vi "GUI Recalculate.vi"(11 "FFmeter settings":T1={"AC Source"={"AC Source type"=enum."Fluke 5XXX calibrator", "VISA"="", "Ref. clock (Hz)"=0.0, "status ref"=refnum}, "TWM pipe"="\\\\.\\pipe\\TWM:server", "Measurement status ref"=refnum, "TWM Status ref"=refnum, "Abort ref"=refnum, "DC meter"={"DC meter type"=enum."H/A/K 3458", "DC meter VISA"="", "NPLC"=10, "No of readings"=3, "status ref"=refnum}, "Measurement properties"={"Measurement frequencies (Hz)"=[1000.0], "Sampling frequency (Hz)"=500000.0, "Signal amplitude (V)"=4.5, "AC-DC settle time (s)"=20.0, "Record length (multiples of period)"=[1000.0, 10000.0, 1000.0], "Measurement template file"=path "", "Row of START keyword"=0, "Row of STOP keyword"=0, "Calculate RMS from samples"=FALSE, "AC-DC warm up time (s)"=300.0, "Measurement template line"=[]}, "Skip waiting ref"=refnum, "Octave paths"={"GNU Octave path"=path "C:/Program Files/GNU Octave/Octave-6.2.0/mingw64/bin", "TWM+QWTB path"=path "C:/Users/labina/Desktop/TWM-1.8.7.0-full/octprog", "lvlib path"=path "D:/martin/WAC/WACsw - github/control_software/Filter function meter/external libraries/GOLPI 0.7.3.1 source distribution LV 20.0 32 bit/lv_proc.dll"}} {"Measurement properties"."Record length (multiples of period)" format="%#_3p"; "Measurement properties"."Sampling frequency (Hz)" format="%#_3p"; "Measurement properties"."Measurement frequencies (Hz)" format="%#_3p"}) -> (3 "FFmeter settings out":T1={"AC Source"={"AC Source type"=enum."Fluke 5XXX calibrator", "VISA"="", "Ref. clock (Hz)"=0.0, "status ref"=refnum}, "TWM pipe"="\\\\.\\pipe\\TWM:server", "Measurement status ref"=refnum, "TWM Status ref"=refnum, "Abort ref"=refnum, "DC meter"={"DC meter type"=enum."H/A/K 3458", "DC meter VISA"="", "NPLC"=10, "No of readings"=3, "status ref"=refnum}, "Measurement properties"={"Measurement frequencies (Hz)"=[1000.0], "Sampling frequency (Hz)"=500000.0, "Signal amplitude (V)"=4.5, "AC-DC settle time (s)"=20.0, "Record length (multiples of period)"=[1000.0, 10000.0, 1000.0], "Measurement template file"=path "", "Row of START keyword"=0, "Row of STOP keyword"=0, "Calculate RMS from samples"=FALSE, "AC-DC warm up time (s)"=300.0, "Measurement template line"=[]}, "Skip waiting ref"=refnum, "Octave paths"={"GNU Octave path"=path "C:/Program Files/GNU Octave/Octave-6.2.0/mingw64/bin", "TWM+QWTB path"=path "C:/Users/labina/Desktop/TWM-1.8.7.0-full/octprog", "lvlib path"=path "D:/martin/WAC/WACsw - github/control_software/Filter function meter/external libraries/GOLPI 0.7.3.1 source distribution LV 20.0 32 bit/lv_proc.dll"}} {"Measurement properties"."Record length (multiples of period)" format="%#_3p"; "Measurement properties"."Sampling frequency (Hz)" format="%#_3p"; "Measurement properties"."Measurement frequencies (Hz)" format="%#_3p"})   [LabVIEW 2020]
doc: "Use this template to build a producer/consumer design pattern with events to produce queue items. Use this design pattern instead of the User Interface Event Handler pattern for user interfaces when you want to execute code asynchronously in response to an event without slowing the user interface responsiveness."
uses:
  GUI/Type definitions/FFmeter settings.ctl
  General AC source/Type definitions/AC Source.ctl
  General AC source/Type definitions/AC Source type.ctl
  General DC meter/Type definitions/DC meter.ctl
  General DC meter/Type definitions/DC meter type.ctl
  Measurement/Type definitions/Measuement properties.ctl
  <vilib>/Utility/NIReport.llb/Report Type.ctl
  external libraries/GOLPI 0.7.3.1 source distribution LV 20.0 32 bit/GOLPI reference Type Def.ctl
  external libraries/GOLPI 0.7.3.1 source distribution LV 20.0 32 bit/Pipe Handle.ctl
  <vilib>/Utility/error.llb/Error Cluster From Error Code.vi
  <vilib>/ErrorRing/Error Ring.xnode
  <vilib>/addons/_office/excel.llb/Excel Get Data ([str]).vi
  external libraries/varilib/varilib.lvlib
  <vilib>/addons/_office/NI_ReportGenerationToolkit.lvlib
  <vilib>/Utility/NIReport.llb/NI_report.lvclass
  <vilib>/Utility/NIReport.llb/NI_ReportGenerationCore.lvlib
  external libraries/GOLPI 0.7.3.1 source distribution LV 20.0 32 bit/LV Process library.lvlib
  external libraries/GOLPI 0.7.3.1 source distribution LV 20.0 32 bit/GOLPI library.lvlib
  <vilib>/Utility/NIReport.llb/Excel/NI_Excel.lvclass
panel:
  out "Progress":i32(slide) min=0 max=3 scale=0.0..10.0
  in  "TWM+QWTB path":path=path "C:/Users/labina/Desktop/TWM-1.8.7.0-full/octprog"
  in  "GNU Octave path":path=path "C:/Program Files/GNU Octave/Octave-6.2.0/mingw64/bin"
  out "gui_elements":refnum<vi>[](array[refnum])
  in  "OK":bool
  in  "cancel":bool
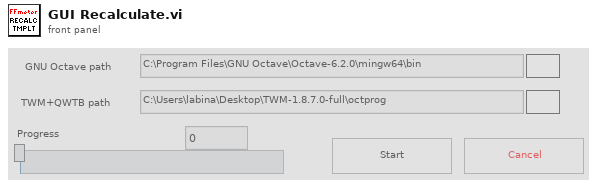
[diagram p1: front panel]
types:
  T1 = typedef "FFmeter settings.ctl" = cluster{"AC Source":T2, "TWM pipe":string, "Measurement status ref":refnum<vi>, "TWM Status ref":refnum<vi>, "Abort ref":refnum<vi>, "DC meter":T4, "Measurement properties":T6, "Skip waiting ref":refnum<vi>, "Octave paths":cluster{"GNU Octave path":path, "TWM+QWTB path":path, "lvlib path":path}}
  T2 = typedef "AC Source.ctl" = cluster{"AC Source type":T3, "VISA":refnum<visa-resource-name>, "Ref. clock (Hz)":dbl, "status ref":refnum<vi>}
  T3 = typedef "AC Source type.ctl" = enum16{"Fluke 5XXX calibrator", "Tektronix AFG3101C", "dummy"}
  T4 = typedef "DC meter.ctl" = cluster{"DC meter type":T5, "DC meter VISA":refnum<visa-resource-name>, "NPLC":i32, "No of readings":i32, "status ref":refnum<vi>}
  T5 = typedef "DC meter type.ctl" = enum16{"H/A/K 3458", "FLuke 8508A", "dummy"}
  T6 = typedef "Measuement properties.ctl" = cluster{"Measurement frequencies (Hz)":dbl[], "Sampling frequency (Hz)":dbl, "Signal amplitude (V)":dbl, "AC-DC settle time (s)":dbl, "Record length (multiples of period)":dbl[], "Measurement template file":path, "Row of START keyword":i32, "Row of STOP keyword":i32, "Calculate RMS from samples":bool, "AC-DC warm up time (s)":dbl, "Measurement template line":i32[]}
  T7 = typedef "GOLPI library.lvlib/GOLPI reference Type Def.ctl" = cluster{"pipe handle":T8, "fast read timeout [ms]":u32, "fast read settle time [ms]":u32, "fast read to multiple [ms]":u32, "max elements per input line":u32, "slow read timeout [ms]":u32, "stdin double format specifier":string, "max elements per stdout output column":u32, "console mode bitstream":bool, "bitstream first read timeout [ms]":u32, "bitstream read timeout [ms]":u32, "struct transfer possible":bool, "matlab mode":bool}
  T8 = typedef "LV Process library.lvlib/Pipe Handle.ctl" = cluster{"lv_proc.dll file path":path, "process instance handle":u32[], "debug mode":bool, "debug data":cluster{"time":timestamp, "stdin":bool, "data":string}[]}
  T9 = enum16{"maximized", "minimized", "normal", "no change"}
  T10 = typedef "NI_ReportGenerationCore.lvlib/Report Type.ctl" = enum16{"HTML", "Word", "Excel"}
  T11 = cluster{"GNU Octave path":path, "TWM+QWTB path":path, "lvlib path":path}
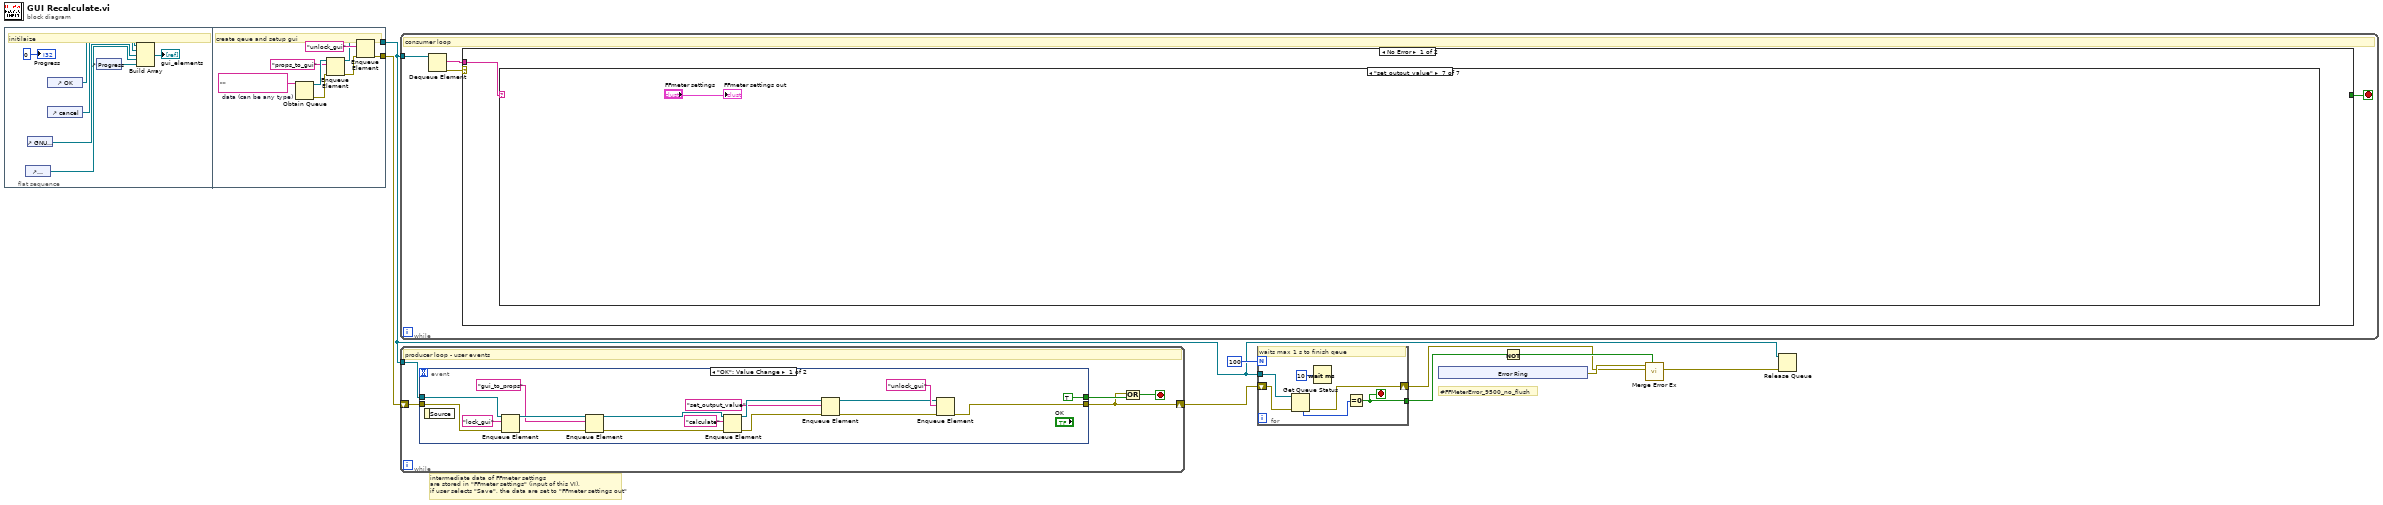
[diagram p0: block diagram]
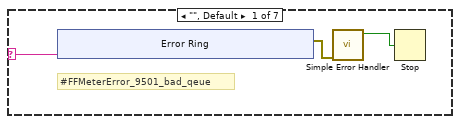
[diagram p2: hidden frame]
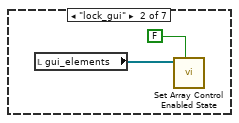
[diagram p3: hidden frame]
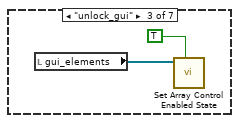
[diagram p4: hidden frame]
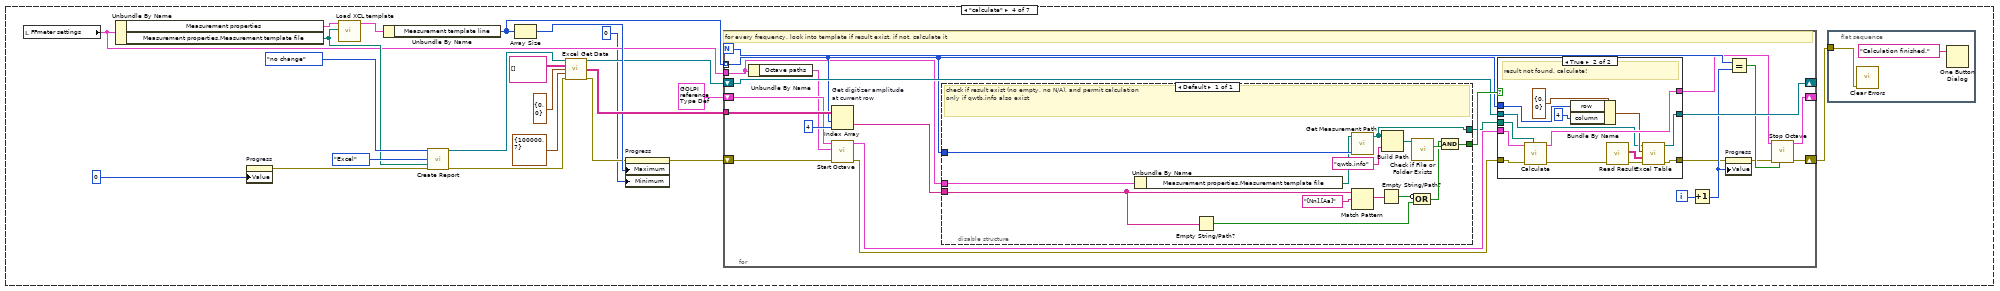
[diagram p5: hidden frame]
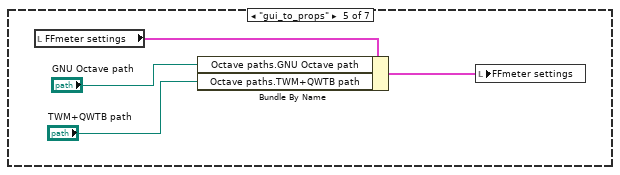
[diagram p7: hidden frame]
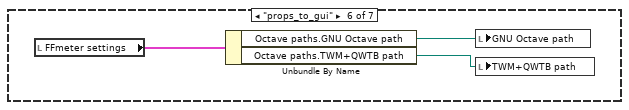
[diagram p8: hidden frame]
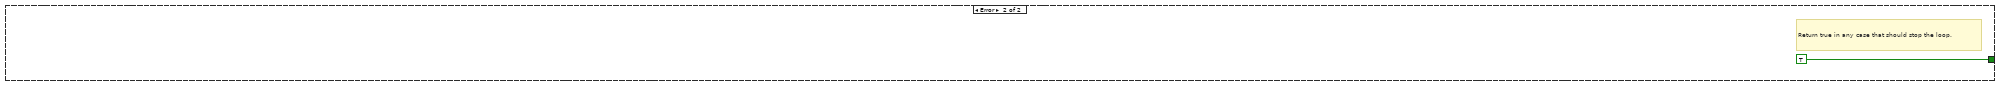
[diagram p9: hidden frame]
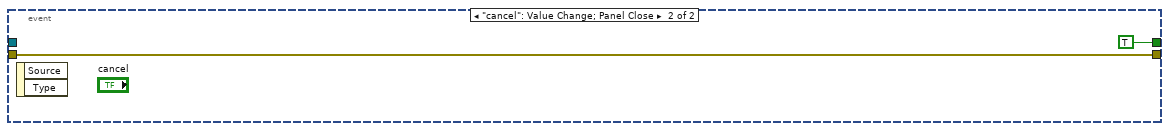
[diagram p10: hidden frame]
diagram:
  # "intermediate data of FFmeter settings\nare stored in \"FFmeter settings\" (input of this VI),\nif user selects \"Save\", the data are set to \"FFmeter settings out\""
  # "#FFMeterError_9500_no_flush"
  n1 = flat-sequence {
    tunnel: [w24] -> w2
    tunnel: [w22] -> w1
    frame #0 {
      # "initilaize"
      n2 = control-ref of="TWM+QWTB path"() -> (w12:refnum<vi>)
      n3 = control-ref of="GNU Octave path"() -> (w13:refnum<vi>)
      n4 = control-ref of="OK"() -> (w16:refnum<vi>)
      n5 = control-ref of="cancel"() -> (w15:refnum<vi>)
      n6 = control-ref of="Progress"() -> (w11:refnum<vi>)
      n7 = Build Array(w16, w15, w13, w12, w11) -> (→"gui_elements":refnum<vi>[])
      "Progress" <- 0 ("Progress")
    }
    frame #1 {
      w23 = ""  # data (can be any type)
      # "create qeue and setup gui"
      n8 = Obtain Queue(element data type=w23) -> (queue out=w19:refnum<queue>, error out=w18:errorcluster)  [unwired: 4 in, 1 out]
      n9 = Enqueue Element(queue=w19, element="props_to_gui", error in (no error)=w18) -> (queue out=w20:refnum<queue>, error out=w21:errorcluster)  [unwired: 1 in, 1 out]
      n10 = Enqueue Element(queue=w20, element="unlock_gui", error in (no error)=w21) -> (queue out=w24:refnum<queue>, error out=w22:errorcluster)  [unwired: 1 in, 1 out]
    }
  }
  n11 = while {
    tunnel: w2 -> [w29]
    stop <- w26 stop-if-true
    # "consumer loop"
    n12 = Dequeue Element(queue=w29) -> (element=w27:string, error out=w28:errorcluster)  [unwired: 2 in, 2 out]
    n13 = case shown="No Error" w28 {
      tunnel: w27 -> [w30 _]
      tunnel: [_ TRUE] -> w26
      frame No Error {
        n14 = case shown="\"set_output_value\"" w30 {
          selector: w30 -> [w31 _ _ _ _ _ _]
          frame "", Default {
            # "#FFMeterError_9501_bad_qeue"
            n15 = xnode "Error Ring"("parameter 0"=w31) -> ("error out"=w33:errorcluster)
            n16 = call <vilib>:"Simple Error Handler.vi"("error in (no error)"=w33) -> ("error?"=w32:bool)  [unwired: 4 in, 4 out]
            n17 = Stop(stop? (T)=w32) -> ()
          }
          frame "lock_gui" {
            n18 = local read "gui_elements"() -> (w42:refnum<vi>[])
            n19 = call "Set Array Control Enabled State.vi"("enabled (T)"=FALSE, "reference array in"=w42) -> ()  [unwired: 8 in, 2 out]
          }
          frame "unlock_gui" {
            n20 = local read "gui_elements"() -> (w44:refnum<vi>[])
            n21 = call "Set Array Control Enabled State.vi"("enabled (T)"=TRUE, "reference array in"=w44) -> ()  [unwired: 8 in, 2 out]
          }
          frame "calculate" {
            n22 = local read "FFmeter settings"() -> (w49:T1)
            n23 = Unbundle By Name(w49) -> ("Measurement properties"=w59:T6, "Measurement properties.Measurement template file"=w56:path)
            n24 = property on="Progress" class="Slide (strict)"("Value"=0 ("Progress")) -> (error out=w53:errorcluster)  [unwired: 2 in, 1 out]
            n25 = call "Load XCL template.vi"("Measurement template file"=w56, "Measurement properties"=w59) -> ("Measurement properties out"=w58:T6)  [unwired: 9 in]
            n26 = Unbundle By Name(w58) -> ("Measurement template line"=w55:i32[])
            n27 = call <vilib>:"Create Report.vi"("window state (normal)"=T9."no change", "report type"=Report_Type."Excel", "template (empty)"=w56, "error in (no error)"=w53) -> ("report out"=w60:refnum<class "NI_report.lvclass">, "error out"=w61:errorcluster)  [unwired: 10 in]
            n28 = Array Size(array=w55) -> (size(s)=w54:i32)
            n29 = call-poly <vilib>:"Excel Get Data.vi"("report in"=w60, "data type"=string[][] [], "start (-1, -1)"=cluster{"row":i32, "column":i32} {"row"=0, "column"=0}, "end (-1, -1)"=cluster{"row":i32, "column":i32} {"row"=100000, "column"=7}, "error in (no error)"=w61) -> ("report out"=w50:refnum<class "NI_report.lvclass">, "data"=w57:string[][], "error out"=w47:errorcluster)  [unwired: 8 in]
            n30 = property on="Progress" class="Slide (strict)"(error in=w47, "Maximum"=w54, "Minimum"=0 ("Data Entry Limits:Minimum")) -> (error out=w46:errorcluster)  [unwired: 1 in, 1 out]
            n31 = for {
              N -> [w85]
              tunnel: w55 -> [w82] mode=indexing
              shift-right: [w75] -> w48
              shift-left: w46 -> [w79]
              tunnel: w57 -> [w91]
              shift-right: [w76] -> _
              shift-left: T7 {"pipe handle"={"lv_proc.dll file path"=path "", "process instance handle"=[], "debug mode"=FALSE, "debug data"=[]}, "fast read timeout [ms]"=500, "fast read settle time [ms]"=10, "fast read to multiple [ms]"=1, "max elements per input line"=100, "slow read timeout [ms]"=5000, "stdin double format specifier"="%_16e", "max elements per stdout output column"=100, "console mode bitstream"=FALSE, "bitstream first read timeout [ms]"=1000, "bitstream read timeout [ms]"=50, "struct transfer possible"=FALSE, "matlab mode"=FALSE} ("GOLPI ref. out") -> [w81]
              shift-right: [w83] -> _
              shift-left: w50 -> [w84]
              tunnel: w49 -> [w72]
              i -> [w86]
              # "for every frequency, look into template if result exist. if not, calculate it"
              n32 = Unbundle By Name(w72) -> ("Octave paths"=w73:T11)
              n33 = Index Array "Get digitizer amplitude\nat current row"(array=w91, index (row)=w82, index (col)=4 ("disabled index (col)")) -> (element=w89:string)
              n34 = call "Start Octave.vi"("error in (no error)"=w79, "Octave paths"=w73, "GOLPI ref. in"=w81) -> ("error out"=w78:errorcluster, "GOLPI ref. out"=w80:T7)  [unwired: 7 in]
              n35 = disable-structure shown="Default" {
                disable-tunnel: w89 -> [w121]
                disable-tunnel: [w112] -> w88
                disable-tunnel: w82 -> [w117]
                disable-tunnel: [w111] -> w87
                disable-tunnel: w72 -> [w110]
                frame Enabled {
                  # "check if result exist (no empty, no N/A), and permit calculation\nonly if qwtb.info also exist"
                  n36 = Unbundle By Name(w110) -> ("Measurement properties.Measurement template file"=w109:path)
                  n37 = Empty String/Path?(string/path=w121) -> (empty?=w118:bool)
                  n38 = call "Get Measurement Path.vi"("Template line"=w117, "Measurement template file"=w109) -> ("Measurement path"=w111:path)  [unwired: 8 in, 1 out]
                  n39 = Match Pattern(string=w121, regular expression="[Nn].[Aa]") -> (match substring=w120:string)  [unwired: 1 in, 3 out]
                  n40 = Empty String/Path?(string/path=w120) -> (empty?=w119:bool)
                  n41 = Build Path(base path=w111, name or relative path="qwtb.info") -> (appended path=w115:path)
                  n42 = call <vilib>:"Check if File or Folder Exists.vi"("path"=w115) -> ("file or folder exists?"=w114:bool)  [unwired: 8 in, 2 out]
                  n43 = Compound Arithmetic op=OR(invert w119, w118) -> (w113:bool)
                  n44 = Compound Arithmetic op=AND(w113, w114) -> (w112:bool)
                }
              }
              n45 = case shown="True" w88 {
                tunnel: [w94 w95] -> w70
                tunnel: w78 -> [w94 w108]
                tunnel: w87 -> [_ w107]
                tunnel: [w93 w106] -> w77
                tunnel: w80 -> [w93 w105]
                tunnel: w84 -> [w92 w101]
                tunnel: [w92 w100] -> w83
                tunnel: w82 -> [_ w99]
                frame False {
                  # "result existr"
                }
                frame True {
                  # "result not found, calculate!"
                  n46 = call "Calculate.vi"("Measurement path in"=w107, "error in (no error)"=w108, "GOLPI ref. in"=w105) -> ("error out"=w104:errorcluster, "GOLPI ref. out"=w106:T7)  [unwired: 7 in]
                  n47 = Bundle By Name(cluster=cluster{"row":i32, "column":i32} {"row"=0, "column"=0} ("start (0, 0)"), "row"=w99, "column"=4) -> (w102:cluster{"row":i32, "column":i32})
                  n48 = call "Read Result.vi"("error in (no error)"=w104) -> ("error out"=w96:errorcluster, "Result (val, unc)"=w97:string[][])  [unwired: 9 in]
                  n49 = call "Excel Table.vi"("error in (no error)"=w96, "table"=w97, "start (0, 0)"=w102, "report in"=w101) -> ("error out"=w95:errorcluster, "report out"=w100:refnum<class "NI_report.lvclass">)  [unwired: 6 in]
                }
              }
              n50 = Increment(x=w86) -> (x+1=w71:i32)
              n51 = property on="Progress" class="Slide (strict)"(error in=w70, "Value"=w71) -> (error out=w69:errorcluster)  [unwired: 1 in, 1 out]
              n52 = Equal?(x=w85, y=w71) -> (x = y?=w74:bool)
              n53 = call "Stop Octave.vi"("Stop Octave?"=w74, "error in (no error)"=w69, "GOLPI ref. in"=w77) -> ("error out"=w75:errorcluster, "GOLPI ref. out"=w76:T7)  [unwired: 7 in]
            }
            n54 = flat-sequence {
              tunnel: w48 -> [w67]
              frame #0 {
                n55 = call <vilib>:"Clear Errors.vi"("error in (no error)"=w67) -> ()  [unwired: 5 in, 2 out]
                n56 = One Button Dialog(message="Calculation finished.") -> ()  [unwired: 1 in, 1 out]
              }
            }
          }
          frame "gui_to_props" {
            n57 = local read "FFmeter settings"() -> (w126:T1)
            n58 = Bundle By Name(cluster=w126, "Octave paths.GNU Octave path"="GNU Octave path", "Octave paths.TWM+QWTB path"="TWM+QWTB path") -> (w125:T1)
            n59 = local write "FFmeter settings"(w125) -> ()
          }
          frame "props_to_gui" {
            n60 = local read "FFmeter settings"() -> (w129:T1)
            n61 = Unbundle By Name(w129) -> ("Octave paths.GNU Octave path"=w127:path, "Octave paths.TWM+QWTB path"=w128:path)
            n62 = local write "GNU Octave path"(w127) -> ()
            n63 = local write "TWM+QWTB path"(w128) -> ()
          }
          frame "set_output_value" {
            "FFmeter settings out" <- "FFmeter settings"
          }
        }
      }
      frame Error {
        # "Return true in any case that should stop the loop."
      }
    }
  }
  n64 = while {
    shift-right: [w132] -> w5
    shift-left: w1 -> [w135]
    tunnel: w2 -> [w136]
    stop <- w133 stop-if-true
    # "producer loop - user events"
    n65 = event shown="[0] \"OK\": Value Change" {
      selector: _ -> [_ _]
      dyn-events: _ -> [_ _]
      timeout: _ -> [_ _]
      tunnel: w136 -> [w150 _]
      tunnel: w135 -> [w149 w155]
      tunnel: [w147 w155] -> w132
      tunnel: [TRUE ("cancel") TRUE ("cancel")] -> w134
      event "OK": Value Change {
        n66 = event-data() -> ()  [unwired: 1 in, 1 out]
        n67 = Enqueue Element(queue=w150, element="lock_gui", error in (no error)=w149) -> (queue out=w143:refnum<queue>, error out=w146:errorcluster)  [unwired: 1 in, 1 out]
        n68 = Enqueue Element(queue=w143, element="gui_to_props", error in (no error)=w146) -> (queue out=w144:refnum<queue>, error out=w145:errorcluster)  [unwired: 1 in, 1 out]
        n69 = Enqueue Element(queue=w144, element="calculate", error in (no error)=w145) -> (queue out=w138:refnum<queue>, error out=w141:errorcluster)  [unwired: 1 in, 1 out]
        n70 = Enqueue Element(queue=w138, element="set_output_value", error in (no error)=w141) -> (queue out=w139:refnum<queue>, error out=w140:errorcluster)  [unwired: 1 in, 1 out]
        n71 = Enqueue Element(queue=w139, element="unlock_gui", error in (no error)=w140) -> (error out=w147:errorcluster)  [unwired: 1 in, 2 out]
      }
      event "cancel": Value Change; Panel Close {
        n72 = event-data() -> ()  [unwired: 1 in, 2 out]
      }
    }
    n73 = Or(x=w132, y=w134) -> (x .or. y?=w133:bool)
  }
  n74 = for {
    N: 100 -> [_]
    tunnel: w2 -> [w161]
    shift-right: [w159] -> w6
    shift-left: w5 -> [w160]
    tunnel: [w156] -> w3
    stop <- w156 stop-if-true
    # "waits max 1 s to finish qeue"
    n75 = Get Queue Status(queue=w161, error in (no error)=w160) -> (error out=w159:errorcluster, # elements in queue=w157:i32)  [unwired: 1 in, 6 out]
    n76 = Wait (ms)(milliseconds to wait=u32 10) -> ()  [unwired: 1 out]
    n77 = Equal To 0?(x=w157) -> (x = 0?=w156:bool)
  }
  n78 = xnode "Error Ring"() -> ("error out"=w7:errorcluster)
  n79 = Not(x=w3) -> (.not. x?=w8:bool)
  n80 = call "Merge Error Ex.vi"("Is error? (False)"=w8, "main error in (no error)"=w6, "second error in"=w7) -> ("error out"=w4:errorcluster)  [unwired: 8 in]
  n81 = Release Queue(queue=w2, error in (no error)=w4) -> ()  [unwired: 1 in, 3 out]
